vi "RelHumToAbsHum.vi"(1 "Temperature (K)":dbl, 2 "Rel. Humidity (%)":dbl) -> (0 "Absolute Humidity (g/m^3)":dbl)   [LabVIEW 2014]
panel:
  out "Constant (g K / J )":dbl=2.16679
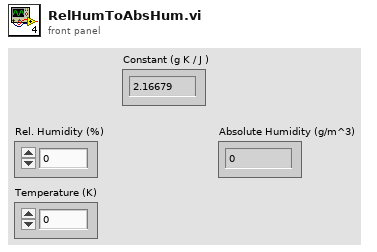
[diagram p1: front panel]
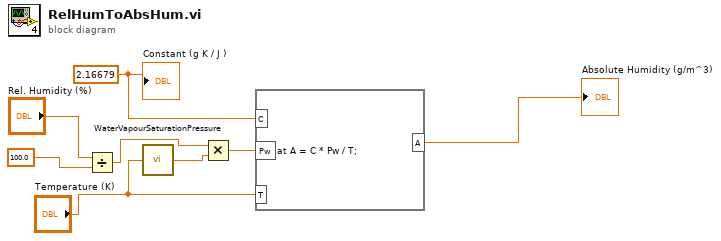
[diagram p0: block diagram]
diagram:
  w2 = 2.16679 ("Constant (g K / J )")
  n1 = Divide(x="Rel. Humidity (%)", y=100.0 ("x")) -> (x/y=w3:dbl)
  n2 = call "WaterVapourSaturationPressure.vi"("Temperature (K)"="Temperature (K)") -> ("Water Vapour Saturation Pressure (Pa)"=w4:dbl)
  n3 = Multiply(x=w3, y=w4) -> (x*y=w5:dbl)
  n4 = formula code="float A = C * Pw / T;"("C"=w2, "Pw"=w5, "T"="Temperature (K)") -> ("A"=→"Absolute Humidity (g/m^3)":dbl)
  "Constant (g K / J )" <- w2
